vi "findVI.vi"(0 "Array":u8[](array[numeric]), 1 "error in (no error)":errorcluster) -> (2 "V":dbl[](array[numeric]), 3 "I":dbl[](array[numeric]), 4 "error out":errorcluster)   [LabVIEW 2016]
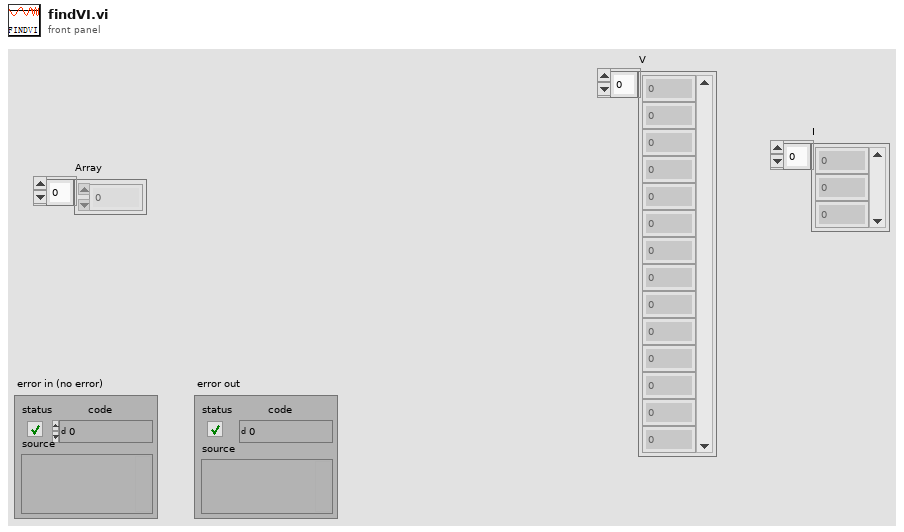
[diagram p1: front panel]
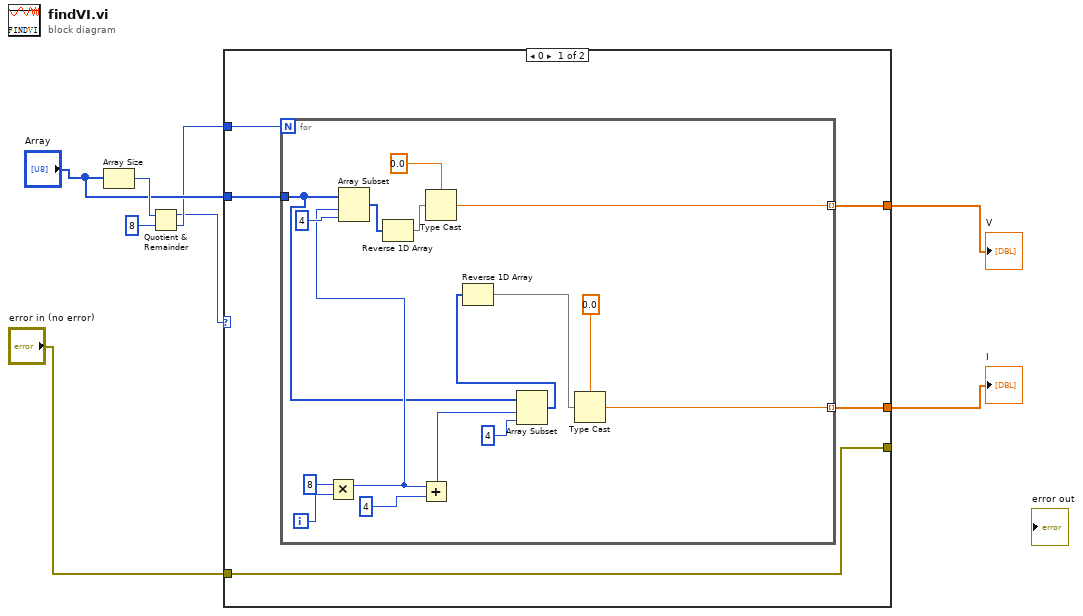
[diagram p0: block diagram]
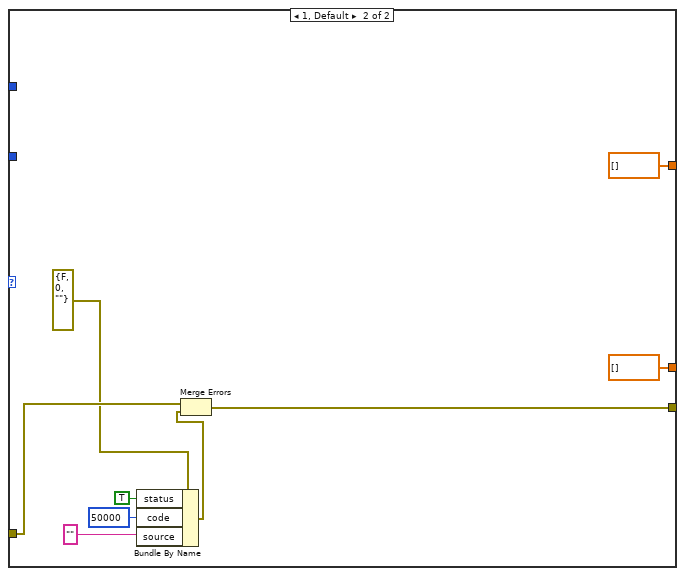
[diagram p2: hidden frame]
diagram:
  n1 = Array Size(array="Array") -> (size(s)=w8:i32)
  n2 = Quotient & Remainder(x=w8, y=8) -> (x-y*floor(x/y)=w1:i32, floor(x/y)=w2:i32)
  n3 = case shown="0" w1 {
    tunnel: "error in (no error)" -> [w10 w38]
    tunnel: [w10 w33] -> _
    tunnel: w2 -> [w13 _]
    tunnel: "Array" -> [w12 _]
    tunnel: [w11 dbl[] []] -> w4
    tunnel: [w9 dbl[] []] -> w3
    frame 0 {
      n4 = for {
        N: w13 -> [_]
        tunnel: w12 -> [w22]
        tunnel: [w25] -> w11 mode=indexing
        tunnel: [w18] -> w9 mode=indexing
        i -> [w29]
        n5 = Multiply(x=8, y=w29) -> (x*y=w24:i32)
        n6 = Array Subset(array=w22, index=w24, length=4) -> (w15:u8[])
        n7 = Reverse 1D Array(array=w15) -> (reversed array=w14:u8[])
        n8 = Add(x=w24, y=4) -> (x+y=w21:i32)
        n9 = Type Cast(type=sgl 0.0, x=w14) -> (*(type *) &x=w25:sgl)
        n10 = Array Subset(array=w22, index=w21, length=4) -> (w17:u8[])
        n11 = Reverse 1D Array(array=w17) -> (reversed array=w16:u8[])
        n12 = Type Cast(type=sgl 0.0, x=w16) -> (*(type *) &x=w18:sgl)
      }
    }
    frame 1, Default {
      n13 = Bundle By Name(cluster=errorcluster {"status"=FALSE, "code"=0, "source"=""} ("error constant"), "status"=TRUE, "code"=50000, "source"="") -> (w34:errorcluster)
      n14 = Merge Errors(w38, w34) -> (w33:errorcluster)
    }
  }
  "V" <- w4
  "I" <- w3
